vi "Vision Processing Tower.vi"(4 "error in (no error)":errorcluster) -> ()   [LabVIEW 2015]
doc: "This VI runs in parallel to other tasks. It gets images from the camera, processes them for color or shape and uses commands or globals to affect the behavior of other subsystems."
uses:
  Support Code/ZMQ Library/zmq_context.lvclass
  Support Code/ZMQ Library/zmq_socket.lvclass
  Support Code/ZMQ Library/socket_type.ctl
  Support Code/ZMQ Library/socket_options.ctl
  <vilib>/Rock Robotics/Network Tables/NT Write Boolean.vi
  Vision Published Globals.vi
  Support Code/ZMQ Library/zeromq.lvlib
panel:
  out "Goal Angle":dbl
  out "Goal Distance":dbl
  out "Goal Detected":bool
  out "context out":refnum<class "zmq_context.lvclass">
  out "data 2":string
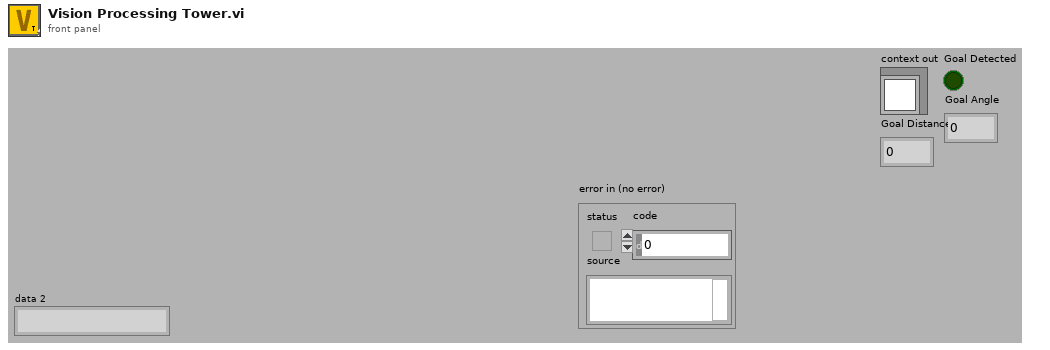
[diagram p1: front panel]
types:
  T1 = typedef "zeromq.lvlib/socket_options.ctl" = enum8{"NONE", "ZMQ_HWM", "<2>", "ZMQ_SWAP", "ZMQ_AFFINITY", "ZMQ_IDENTITY", "ZMQ_SUBSCRIBE", "ZMQ_UNSUBSCRIBE", "ZMQ_RATE", "ZMQ_RECOVERY_IVL", "ZMQ_MCAST_LOOP", "ZMQ_SNDBUF", "ZMQ_RCVBUF", "ZMQ_RCVMORE", "ZMQ_FD", "ZMQ_EVENTS", "ZMQ_TYPE", "ZMQ_LINGER", "ZMQ_RECONNECT_IVL", "ZMQ_BACKLOG", "ZMQ_RECOVERY_IVL_MSEC", "ZMQ_RECONNECT_IVL_MAX", "ZMQ_MAXMSGSIZE", "ZMQ_SNDHWM", "ZMQ_RCVHWM", "ZMQ_MULTICAST_HOPS", "<26>", "ZMQ_RCVTIMEO", "ZMQ_SNDTIMEO", "<29>", "<30>", "ZMQ_IPV4ONLY", "ZMQ_LAST_ENDPOINT", "ZMQ_ROUTER_MANDATORY", "ZMQ_TCP_KEEPALIVE", "ZMQ_TCP_KEEPALIVE_CNT", "ZMQ_TCP_KEEPALIVE_IDLE", "ZMQ_TCP_KEEPALIVE_INTVL", "ZMQ_TCP_ACCEPT_FILTER", "ZMQ_DELAY_ATTACH_ON_CONNECT", "ZMQ_XPUB_VERBOSE"}
  T2 = typedef "zeromq.lvlib/socket_type.ctl" = enum8{"ZMQ_PAIR", "ZMQ_PUB", "ZMQ_SUB", "ZMQ_REQ", "ZMQ_REP", "ZMQ_DEALER", "ZMQ_ROUTER", "ZMQ_PULL", "ZMQ_PUSH", "ZMQ_XPUB", "ZMQ_XSUB"}
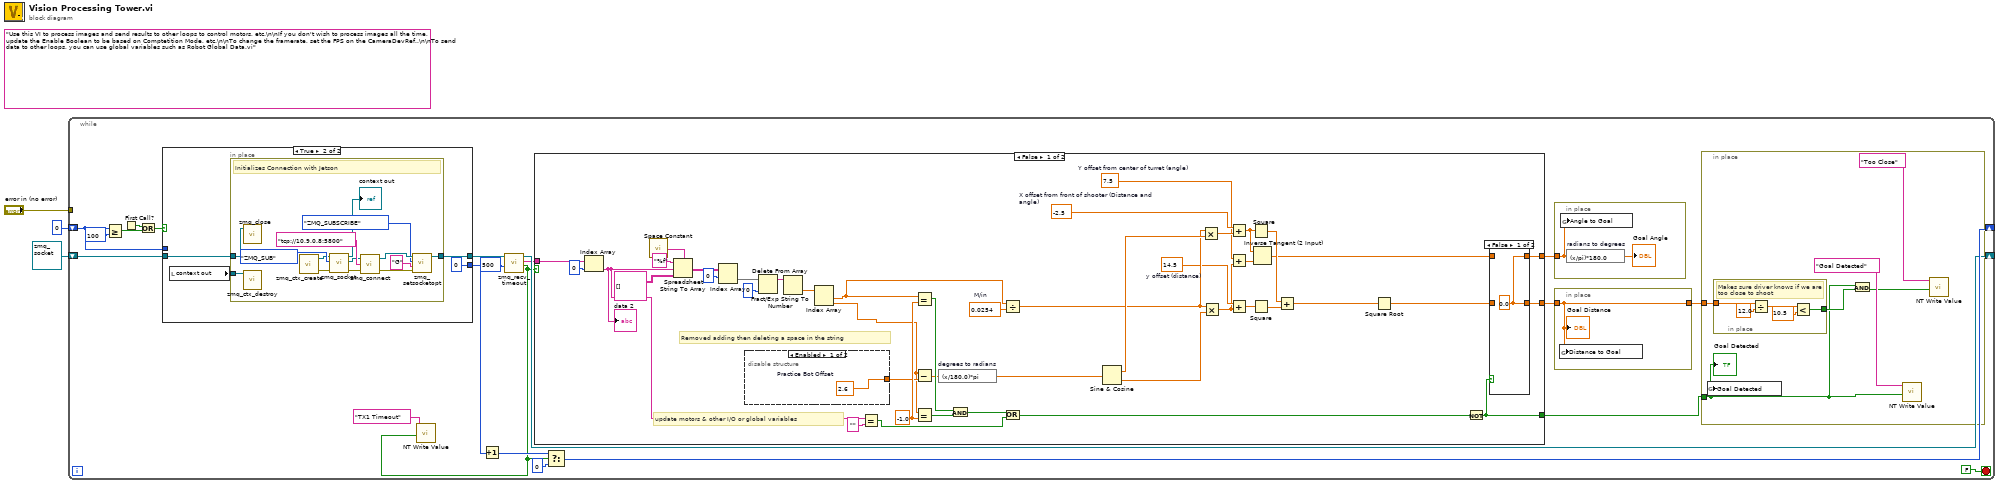
[diagram p0: block diagram]
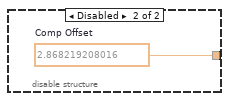
[diagram p2: hidden frame]
diagram:
  (unwired) "Use this VI to process images and send results to other loops to control motors, etc.\n\nIf you don't wish to process images all the time, update the Enable Boolean to be based on Comptetition Mode, etc.\n\nTo change the framerate, set the FPS on the CameraDevRef..\n\nTo send data to other loops, you can use global variables such as Robot Global Data.vi"
  n1 = while {
    tunnel: "error in (no error)" -> [_]
    shift-right: [w14] -> _
    shift-left: refnum<class "zmq_socket.lvclass"> refnum ("socket out") -> [w15]
    shift-right: [w23] -> _
    shift-left: 0 -> [w17]
    stop <- FALSE stop-if-true
    n2 = Greater Or Equal?(x=w17, y=100) -> (x >= y?=w21:bool)
    n3 = First Call?() -> (First Call?: T/F=w19:bool)
    n4 = Or(x=w19, y=w21) -> (x .or. y?=w20:bool)
    n5 = case shown="True" w20 {
      tunnel: [w89 0] -> w18
      tunnel: w17 -> [w89 _]
      tunnel: [w88 w92] -> w16
      tunnel: w15 -> [w88 w91]
      frame False {
      }
      frame True {
        n6 = local read "context out"() -> (w90:refnum<class "zmq_context.lvclass">)
        n7 = in-place {
          in-place-border: [w97] -> w92
          in-place-border: w91 -> [w94]
          in-place-border: w90 -> [w95]
          # "Initializes Connection with Jetson"
          n8 = call "zmq_close.vi"("socket"=w94) -> ()  [unwired: 4 in, 1 out]
          n9 = call "zmq_ctx_destroy.vi"("context in"=w95) -> ()  [unwired: 4 in, 1 out]
          n10 = call "zmq_ctx_create.vi"() -> ("error out"=w105:errorcluster, "context out"=w106:refnum<class "zmq_context.lvclass">)  [unwired: 4 in]
          n11 = call "zmq_socket.vi"("error in"=w105, "socket type"=socket_type."ZMQ_SUB", "context in"=w106) -> ("error out"=w102:errorcluster, "socket out"=w103:refnum<class "zmq_socket.lvclass">, "context out"=→"context out":refnum<class "zmq_context.lvclass">)  [unwired: 2 in]
          n12 = call "zmq_connect.vi"("error in"=w102, "endpoint"="tcp://10.9.0.8:5800" ("Endpoint"), "socket in"=w103) -> ("error out"=w99:errorcluster, "socket out"=w100:refnum<class "zmq_socket.lvclass">)  [unwired: 1 in]
          n13 = call "zmq_setsocketopt.vi"("error in"=w99, "value"="G", "option"=socket_options."ZMQ_SUBSCRIBE", "socket in"=w100) -> ("socket out"=w97:refnum<class "zmq_socket.lvclass">)  [unwired: 2 in, 1 out]
        }
      }
    }
    n14 = Increment(x=w18) -> (x+1=w11:i32)
    n15 = call "zmq_recv_timeout.vi"("timeout (ms)"=u32 500, "socket in"=w16) -> ("timeout?"=w4:bool, "parts"=w12:string[], "socket out"=w14:refnum<class "zmq_socket.lvclass">)  [unwired: 2 in, 1 out]
    n16 = call-poly <vilib>:"NT Write Value.vi"("Boolean"=w4, "Name"="TX1 Timeout") -> ()  [unwired: 9 in, 1 out]
    n17 = case shown="False" w4 {
      tunnel: w12 -> [w52 _]
      tunnel: [w46 _] -> w9
      tunnel: [w45 _] -> w8
      tunnel: [w44 _] -> w7
      frame False {
        w48 = 7.5  # Y offset from center of turret (angle)
        w71 = 14.5  # y offset (distance)
        w72 = -2.5  # X offset from front of shooter (Distance and angle)
        w82 = 0.0254  # M/in
        w65 = -1.0 ("y")
        # "Removed adding then deleting a space in the string"
        # "update motors & other I/O or global variables"
        n18 = Index Array(array=w52, index=0) -> (element=w41:string)
        "data 2" <- w41
        n19 = call <vilib>:"Space Constant.vi"() -> ("String"=w58:string)
        n20 = Spreadsheet String To Array(delimiter (Tab)=w58, format string="%f", spreadsheet string=w41, array type (2D Dbl)=string[][] [] ("Array")) -> (array=w40:string[][])
        n21 = Index Array(array=w40, index (row)=0) -> (element=w55:string[])  [unwired: 1 in]
        n22 = disable-structure shown="Enabled" {
          disable-tunnel: [w83 w84] -> w43
          frame Enabled {
            w83 = 2.6  # Practice Bot Offset
          }
          frame Disabled {
            w84 = 2.868219208016  # Comp Offset
          }
        }
        n23 = Delete From Array(array=w55, index=0) -> (array with subset deleted=w54:string[])  [unwired: 1 in, 1 out]
        n24 = Fract/Exp String To Number(string=w54) -> (number=w51:dbl[])  [unwired: 4 out]
        n25 = Index Array(array=w51) -> (element #1=w61:dbl, element #2=w39:dbl)  [unwired: 2 in]
        n26 = Equal?(x=w41, y="") -> (x = y?=w69:bool)
        n27 = Equal?(x=w61, y=w65) -> (x = y?=w63:bool)
        n28 = Subtract(x=w39, y=w43) -> (x-y=w42:dbl)
        n29 = Equal?(x=w39, y=w65) -> (x = y?=w64:bool)
        n30 = expression code="(x/180.0)*pi" "degrees to radians"(w42) -> (w81:dbl)
        n31 = And(x=w63, y=w64) -> (x .and. y?=w62:bool)
        n32 = Divide(x=w61, y=w82) -> (x/y=w78:dbl)
        n33 = Or(x=w62, y=w69) -> (x .or. y?=w68:bool)
        n34 = Sine & Cosine(0:w81) -> (1:w80:dbl, 2:w50:dbl)
        n35 = Multiply(x=w78, y=w80) -> (x*y=w79:dbl)
        n36 = Multiply(x=w78, y=w50) -> (x*y=w47:dbl)
        n37 = Add(x=w72, y=w79) -> (x+y=w74:dbl)
        n38 = Add(x=w48, y=w47) -> (x+y=w49:dbl)
        n39 = Add(x=w71, y=w47) -> (x+y=w73:dbl)
        n40 = Square(x=w74) -> (x^2=w77:dbl)
        n41 = Square(x=w73) -> (x^2=w76:dbl)
        n42 = Inverse Tangent (2 Input)(1:w49, 2:w74) -> (0:w67:dbl)
        n43 = Add(x=w77, y=w76) -> (x+y=w75:dbl)
        n44 = Square Root(x=w75) -> (sqrt(x)=w66:dbl)
        n45 = Not(x=w68) -> (.not. x?=w44:bool)
        n46 = case shown="False" w44 {
          tunnel: [w85 w87] -> w46
          tunnel: w67 -> [_ w87]
          tunnel: [w85 w86] -> w45
          tunnel: w66 -> [_ w86]
          frame False {
            w85 = 0.0
          }
          frame True {
          }
        }
      }
      frame True {
      }
    }
    n47 = Select(t=w11, s=w4, f=0) -> (s? t:f=w23:i32)
    n48 = in-place {
      in-place-border: w9 -> [w27]
      n49 = global write "Vision Published Globals.vi" "Angle to Goal"(w27) -> ()
      n50 = expression code="(x/pi)*180.0" "radians to degrees"(w27) -> (→"Goal Angle":dbl)
    }
    n51 = in-place {
      in-place-border: w8 -> [w25]
      in-place-border: [w25] -> w6
      n52 = global write "Vision Published Globals.vi" "Distance to Goal"(w25) -> ()
      "Goal Distance" <- w25
    }
    n53 = in-place {
      in-place-border: w7 -> [w28]
      in-place-border: w6 -> [w32]
      n54 = global write "Vision Published Globals.vi" "Goal Detected"(w28) -> ()
      n55 = in-place {
        in-place-border: w32 -> [w37]
        in-place-border: [w34] -> w30
        # "Makes sure driver knows if we are too close to shoot"
        n56 = Divide(x=w37, y=12.0) -> (x/y=w36:dbl)
        n57 = Less?(x=w36, y=10.5) -> (x < y?=w34:bool)
      }
      n58 = And(x=w28, y=w30) -> (x .and. y?=w29:bool)
      n59 = call-poly <vilib>:"NT Write Value.vi"("Boolean"=w28, "Name"="Goal Detected") -> ()  [unwired: 9 in, 1 out]
      n60 = call-poly <vilib>:"NT Write Value.vi"("Boolean"=w29, "Name"="Too Close") -> ()  [unwired: 9 in, 1 out]
      "Goal Detected" <- w28
    }
  }
